vi "Playback.vi"(8 "stop":bool, 10 "Volume":dbl(slide) scale=0.0..10.0, 11 "file path (dialog if empty)":path) -> (2 "Waveform Graph":waveform(dbl)[](graph))   [LabVIEW 2014]
uses:
  <vilib>/Waveform/WDTFileIO.llb/Read Waveform from File.vi
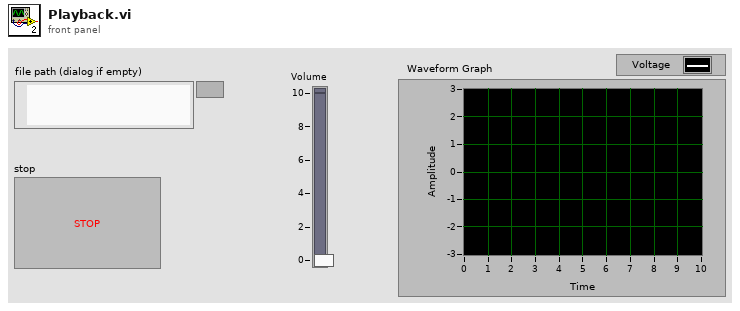
[diagram p1: front panel]
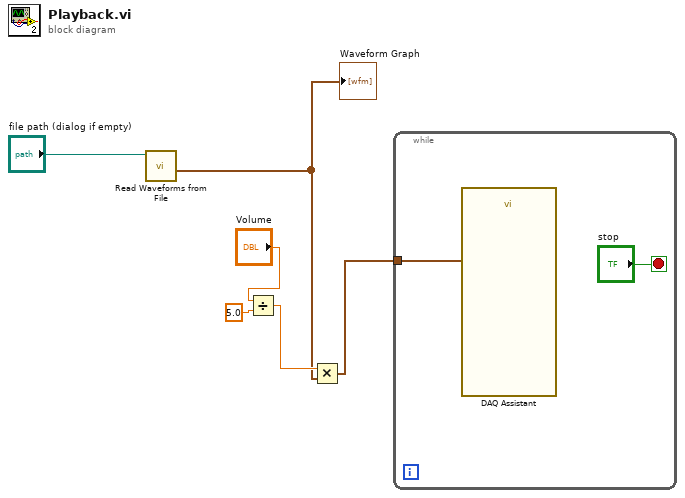
[diagram p0: block diagram]
diagram:
  n1 = call-poly <vilib>:"Read Waveforms from File.vi"("file path (dialog if empty)"="file path (dialog if empty)") -> ("all waveforms in record"=w1:waveform(dbl)[])  [unwired: 5 in, 3 out]
  "Waveform Graph" <- w1
  n2 = Divide(x="Volume", y=5.0) -> (x/y=w4:dbl)
  n3 = Multiply(x=w4, y=w1) -> (x*y=w2:waveform(dbl)[])
  n4 = while {
    tunnel: w2 -> [w8]
    stop <- "stop" stop-if-true
    n5 = call "DAQ Assistant"("data"=w8) -> ()  [unwired: 16 in, 3 out]
  }
